vi "writeI24.vi"(8 "error in (no error)":errorcluster, 10 "Input":i32, 11 "ModbusBuffer in":refnum<class "ModbusBuffer.lvclass">) -> (0 "error out":errorcluster, 3 "ModbusBuffer out":refnum<class "ModbusBuffer.lvclass">)   [LabVIEW 2016, in "RTModbus.lvlib" / "ModbusBuffer.lvclass"]
uses:
  ModbusBuffer.lvclass
  ModbusBuffer.lvclass/ModbusBuffer.ctl
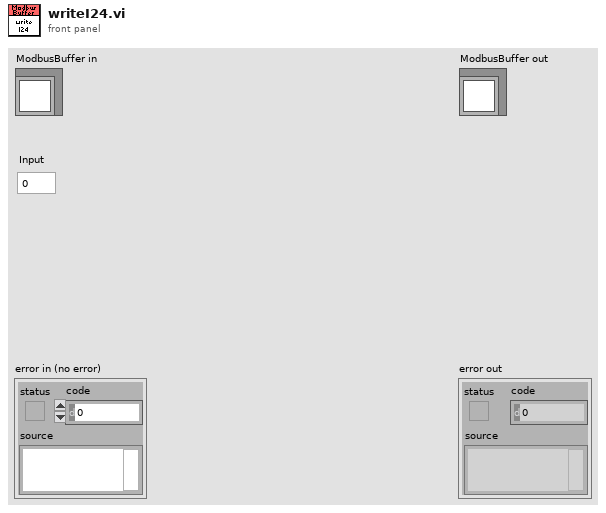
[diagram p1: front panel]
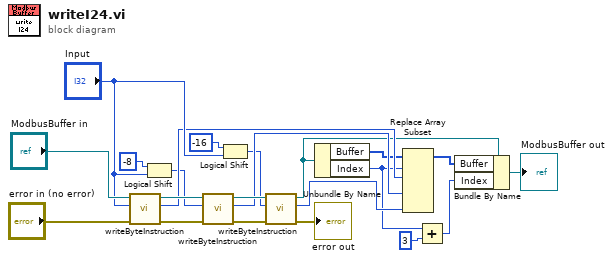
[diagram p0: block diagram]
diagram:
  n1 = call "writeByteInstruction.vi"("error in (no error)"="error in (no error)", "Input"="Input", "ModbusBuffer in"="ModbusBuffer in") -> ("error out"=w7:errorcluster, "Output"=w13:u16, "ModbusBuffer out"=w16:refnum<class "ModbusBuffer.lvclass">)  [unwired: 6 in]
  n2 = Logical Shift(y=i16 -8, x="Input") -> (x << y=w11:i32)
  n3 = call "writeByteInstruction.vi"("error in (no error)"=w7, "Input"=w11, "ModbusBuffer in"=w16) -> ("error out"=w6:errorcluster, "Output"=w12:u16, "ModbusBuffer out"=w15:refnum<class "ModbusBuffer.lvclass">)  [unwired: 6 in]
  n4 = Logical Shift(y=i16 -16, x="Input") -> (x << y=w10:i32)
  n5 = call "writeByteInstruction.vi"("error in (no error)"=w6, "Input"=w10, "ModbusBuffer in"=w15) -> ("error out"=→"error out":errorcluster, "Output"=w9:u16, "ModbusBuffer out"=w5:refnum<class "ModbusBuffer.lvclass">)  [unwired: 6 in]
  n6 = Unbundle By Name(w5) -> ("Buffer"=w3:u16[], "Index"=w2:i32)
  n7 = Replace Array Subset(array=w3, new element #1=w13, index #1=w2, new element #2=w12, new element #3=w9) -> (w18:u16[])  [unwired: 2 in]
  n8 = Add(x=w2, y=3) -> (x+y=w21:i32)
  n9 = Bundle By Name(cluster=w5, "Buffer"=w18, "Index"=w21) -> (→"ModbusBuffer out":refnum<class "ModbusBuffer.lvclass">)
